vi "Sub_Get_Number_from_Remaining_Length.vi"(8 "error in (no error)":errorcluster, 10 "Remaining Length":u8[](array[numeric]) format="%x", 11 "SSL_Connection":T1) -> (0 "error out":errorcluster, 2 "X":u32, 3 "SSL_Connection":T1)   [LabVIEW 2015]
uses:
  Controls/SSL_Connection.ctl
  AWS_IoT.lvlib
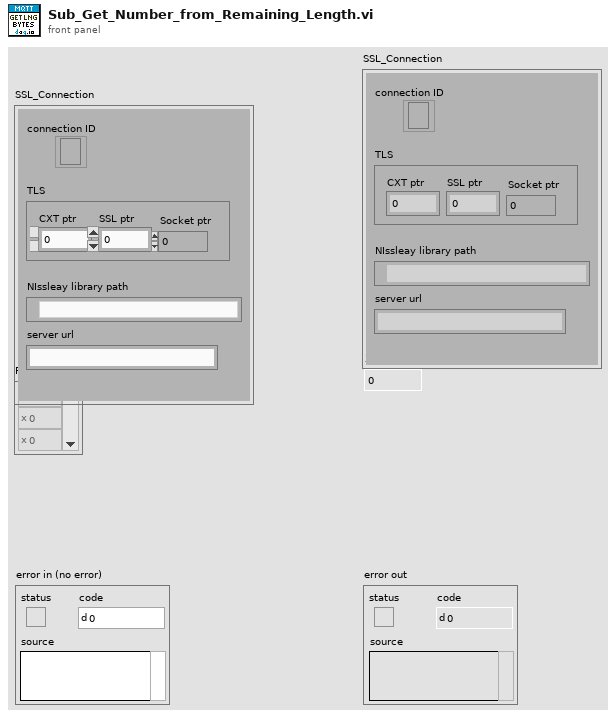
[diagram p1: front panel]
types:
  T1 = typedef "AWS_IoT.lvlib/SSL_Connection.ctl" = cluster{"connection ID":refnum<k5>, "TLS":cluster{"CXT ptr":i32, "SSL ptr":i32, "Socket ptr":i32}, "NIssleay library path":path, "server url":string}
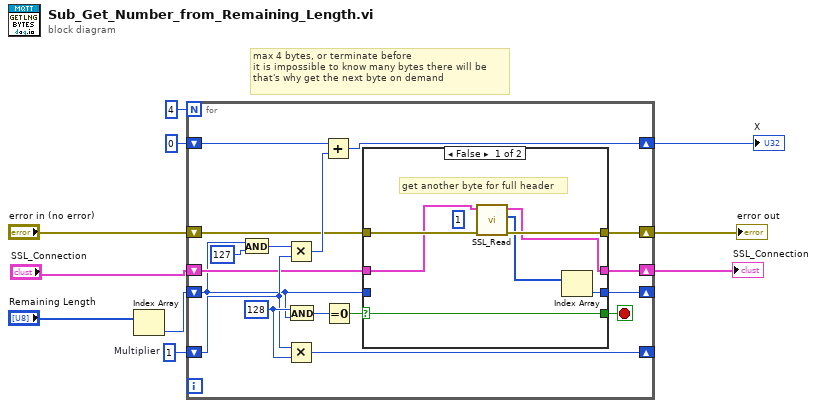
[diagram p0: block diagram]
diagram:
  w10 = u32 1  # Multiplier
  # "max 4 bytes, or terminate before\nit is impossible to know many bytes there will be\nthat's why get the next byte on demand"
  n1 = Index Array(array="Remaining Length") -> (element=w3:u8)  [unwired: 1 in]
  n2 = for {
    N: 4 -> [_]
    shift-right: [w27] -> _
    shift-left: w10 -> [w20]
    shift-right: [w22] -> w8
    shift-left: u32 0 -> [w24]
    shift-right: [w14] -> w5
    shift-left: "error in (no error)" -> [w15]
    shift-right: [w13] -> _
    shift-left: w3 -> [w12]
    shift-right: [w11] -> w1
    shift-left: "SSL_Connection" -> [w16]
    stop <- w17 stop-if-true
    w21 = u32 128 ("y")
    n3 = And(x=w12, y=u8 127) -> (x .and. y?=w25:u8)
    n4 = Multiply(x=w25, y=w20) -> (x*y=w23:u32)
    n5 = Multiply(x=w20, y=w21) -> (x*y=w27:u32)
    n6 = And(x=w21, y=w12) -> (x .and. y?=w19:u32)
    n7 = Add(x=w24, y=w23) -> (x+y=w22:u32)
    n8 = Equal To 0?(x=w19) -> (x = 0?=w18:bool)
    n9 = case shown="False" w18 {
      selector: w18 -> [w34 w38]
      tunnel: [w34 w38] -> w17
      tunnel: w16 -> [w30 w35]
      tunnel: w15 -> [w33 w37]
      tunnel: [w32 w37] -> w14
      tunnel: [w31 w36] -> w13
      tunnel: w12 -> [_ w36]
      tunnel: [w29 w35] -> w11
      frame False {
        (unwired) 1 ("bytes to read")
        # "get another byte for full header"
        n10 = call "SSL_Read.vi"("error in (no error)"=w33, "SSL_Connection"=w30) -> ("error out"=w32:errorcluster, "data out"=w28:u8[], "SSL_Connection 2"=w29:T1)  [unwired: 6 in, 1 out]
        n11 = Index Array(array=w28) -> (element=w31:u8)  [unwired: 1 in]
      }
      frame True {
      }
    }
  }
  "error out" <- w5
  "X" <- w8
  "SSL_Connection" <- w1
